vi "user32_GetCursorPos.vi"(11 "错误输入（无错误）":errorcluster) -> (15 "错误输出":errorcluster)   [LabVIEW 2013]
doc: "该函数分配一个新菜单到指定窗口。"
uses:
  user32.dll
panel:
  out "Position":cluster{"x":i32, "y":i32}
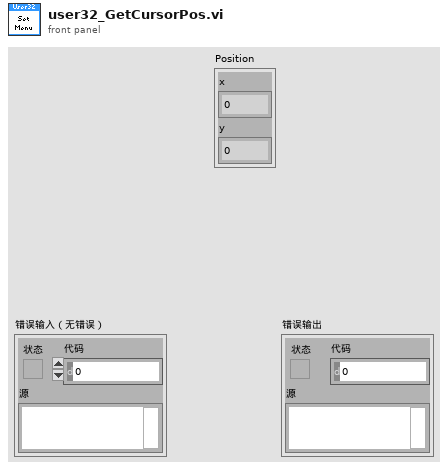
[diagram p1: front panel]
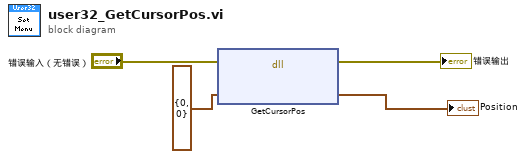
[diagram p0: block diagram]
diagram:
  n1 = dll-call lib="user32.dll" fn="GetCursorPos"(error in="错误输入（无错误）", "Position"=cluster{"x":i32, "y":i32} {"x"=0, "y"=0}) -> (error out=→"错误输出":errorcluster, "Position"=→"Position":cluster{"x":i32, "y":i32})  [unwired: 3 in, 1 out]
